vi "JSON_Metadata_Test.vi"() -> ()   [LabVIEW 2016]
uses:
  METADATA.ctl
panel:
  out "Sweeping Infos":T1(array[cluster])
  out "concatenated string":string
  out "data":T2
  in  "Metadata Cluster":T2
  in  "JSON destination":path
  out "JSON String":string
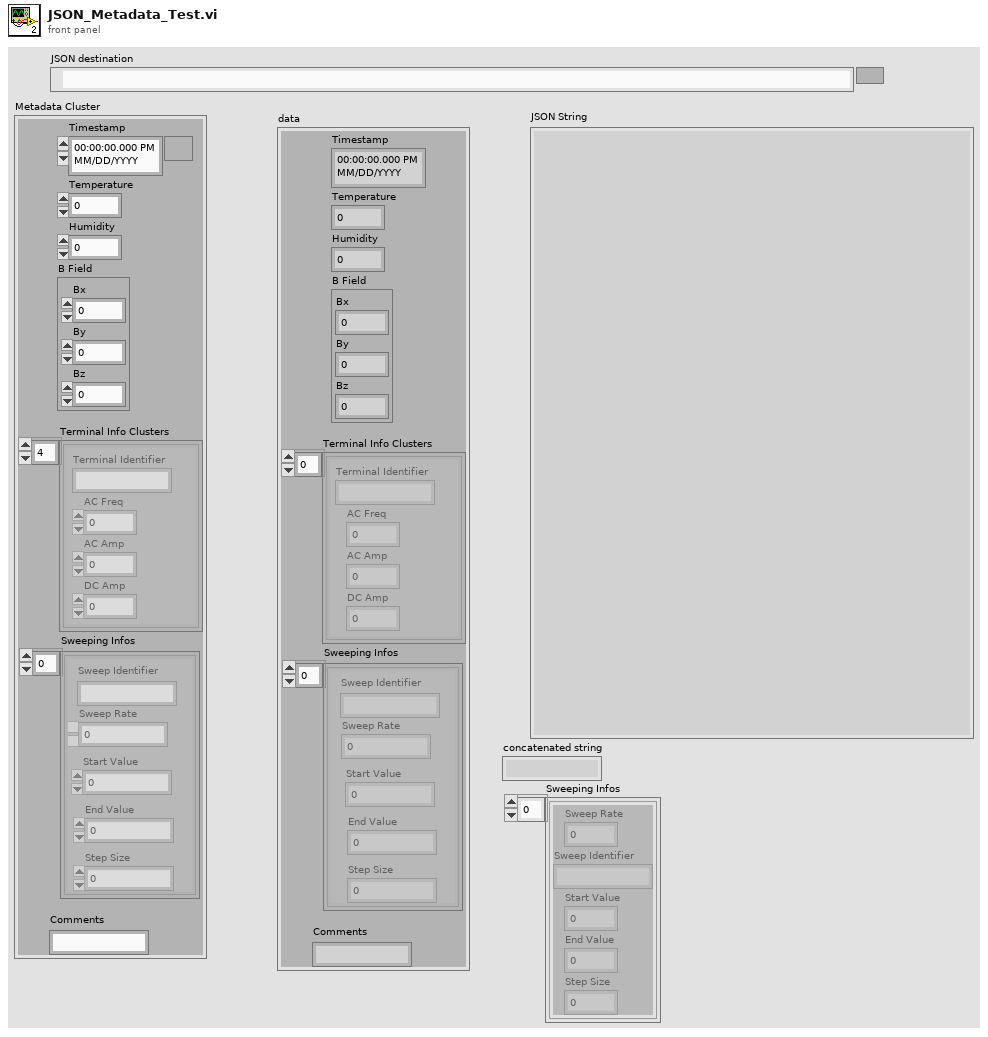
[diagram p1: front panel]
types:
  T1 = cluster{"Sweep Rate":dbl, "Sweep Identifier":string, "Start Value":dbl, "End Value":dbl, "Step Size":dbl}[]
  T2 = typedef "METADATA.ctl" = cluster{"Timestamp":timestamp, "Temperature":dbl, "Humidity":dbl, "B Field":cluster{"Bx":dbl, "By":dbl, "Bz":dbl}, "Terminal Info Clusters":cluster{"Terminal Identifier":string, "AC Freq":dbl, "AC Amp":dbl, "DC Amp":dbl}[], "Sweeping Infos":cluster{"Sweep Rate":dbl, "Sweep Identifier":string, "Start Value":dbl, "End Value":dbl, "Step Size":dbl}[], "Comments":string}
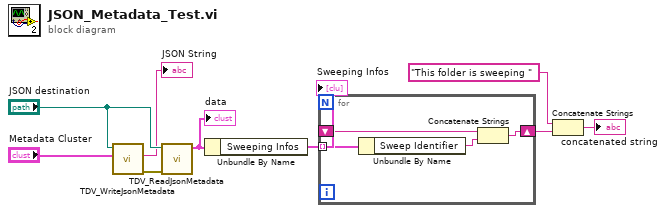
[diagram p0: block diagram]
diagram:
  n1 = call "TDV_WriteJsonMetadata.vi"("Metadata Cluster"="Metadata Cluster", "JSON destination"="JSON destination") -> ("error out"=w3:errorcluster, "JSON String"=→"JSON String":string)  [unwired: 6 in, 2 out]
  n2 = call "TDV_ReadJsonMetadata.vi"("error in (no error)"=w3, "JSON Source"="JSON destination") -> ("METADATA"=w2:T2)  [unwired: 8 in, 1 out]
  "data" <- w2
  n3 = Unbundle By Name(w2) -> ("Sweeping Infos"=w9:T1)
  "Sweeping Infos" <- w9
  n4 = for {
    tunnel: w9 -> [w11] mode=indexing
    shift-right: [w13] -> w7
    shift-left: _ -> [w12]
    n5 = Unbundle By Name(w11) -> ("Sweep Identifier"=w10:string)
    n6 = Concatenate Strings(w12, w10) -> (w13:string)
  }
  n7 = Concatenate Strings("This folder is sweeping " ("string"), w7) -> (→"concatenated string":string)
